vi "Untitled 1.vi"   [LabVIEW 2012]
uses:
  <vilib>/Distrio/Murmex/GenericMessage/GenericMessage.lvclass
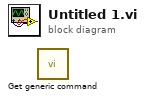
[diagram p0: block diagram]
diagram:
  n1 = call <vilib>:"Get generic command.vi"() -> ()  [unwired: 9 in, 3 out]
